vi "Analog Input Engine.vi"(5 "Main Engine Q":refnum<queue>, 7 "TCP Enigine Q":refnum<queue>, 8 "error in":errorcluster, 10 "Engine Name":string, 11 "Varient Data":variant) -> (0 "error out":errorcluster)   [LabVIEW 2024]
doc: "All Rights Reserved © 2023 SyncSols"
uses:
  Controls/Analog Input SM Data Cluster.ctl
  Analog Output/Controls/AIO Command Q Cluster.ctl
  Analog Output/Controls/AO Interface Data Cluster.ctl
  Analog Output/Controls/AO Channel Configuration Cluster.ctl
  Analog Output/Controls/AO Timing Cluster.ctl
  Main Engine/Controls/Main Engine JSON Command State.ctl
  TCP Engine/Controls/TCP Engine I&O  Interupt Cluster.ctl
  Host-DQMH/Configuration/Analog Input Single Channel Data--Cluster.ctl
  Host-DQMH/Configuration/Config-Channel Type.ctl
  Host-DQMH/Configuration/Channel Sub-Type.ctl
  Controls/Analog Input SM Cases.ctl
  Main Engine/Controls/Main Engine Engine No.Options.ctl
  Host-DQMH/Configuration/All Interface Data.ctl
  Host-DQMH/Configuration/DO Channel's.ctl
  Analog Output/Controls/AO JSON Data Cluster.ctl
  Main Engine/Controls/Main Engine Config Confirmation Cluster.ctl
  TCP Engine/TCP Engine.lvlib
  Host-DQMH/Configuration/Configuration.lvlib
panel:
  out "error out 4":errorcluster
  out "error out 3":errorcluster
  out "error out 2":errorcluster
  out "Configuration Data":T1[](array[typedef])
  in  "Data Cluster":T2={"TCP Engine Response Q"=refnum, "Main Engine Response Q"=refnum, "Command Q"=refnum, "Interupt Q"=refnum, "Stop Notifier"=refnum, "Start Notifier"=refnum, "Varient Data"=variant(string ""), "Engine Name"="", "Configuration Data"=[], "AI Task"="", "Single Sample?"=FALSE, "AI Config Data"={"Module Name"="", "AI Channel's Data"=[], "Analog Input Timing"={"samples per channel"=0, "sample mode"=0, "Sampling Rate"=0.0}}, "Configured Data's"={"Channel Names"=[], "Identification Names"=[]}, "AI Log File Path"=path ""} {"AI Config Data"."Analog Input Timing"."sample mode" items=["Finite Samples"=10178, "Continuous Samples"=10123, "Hardware Timed Single Point"=12522]}
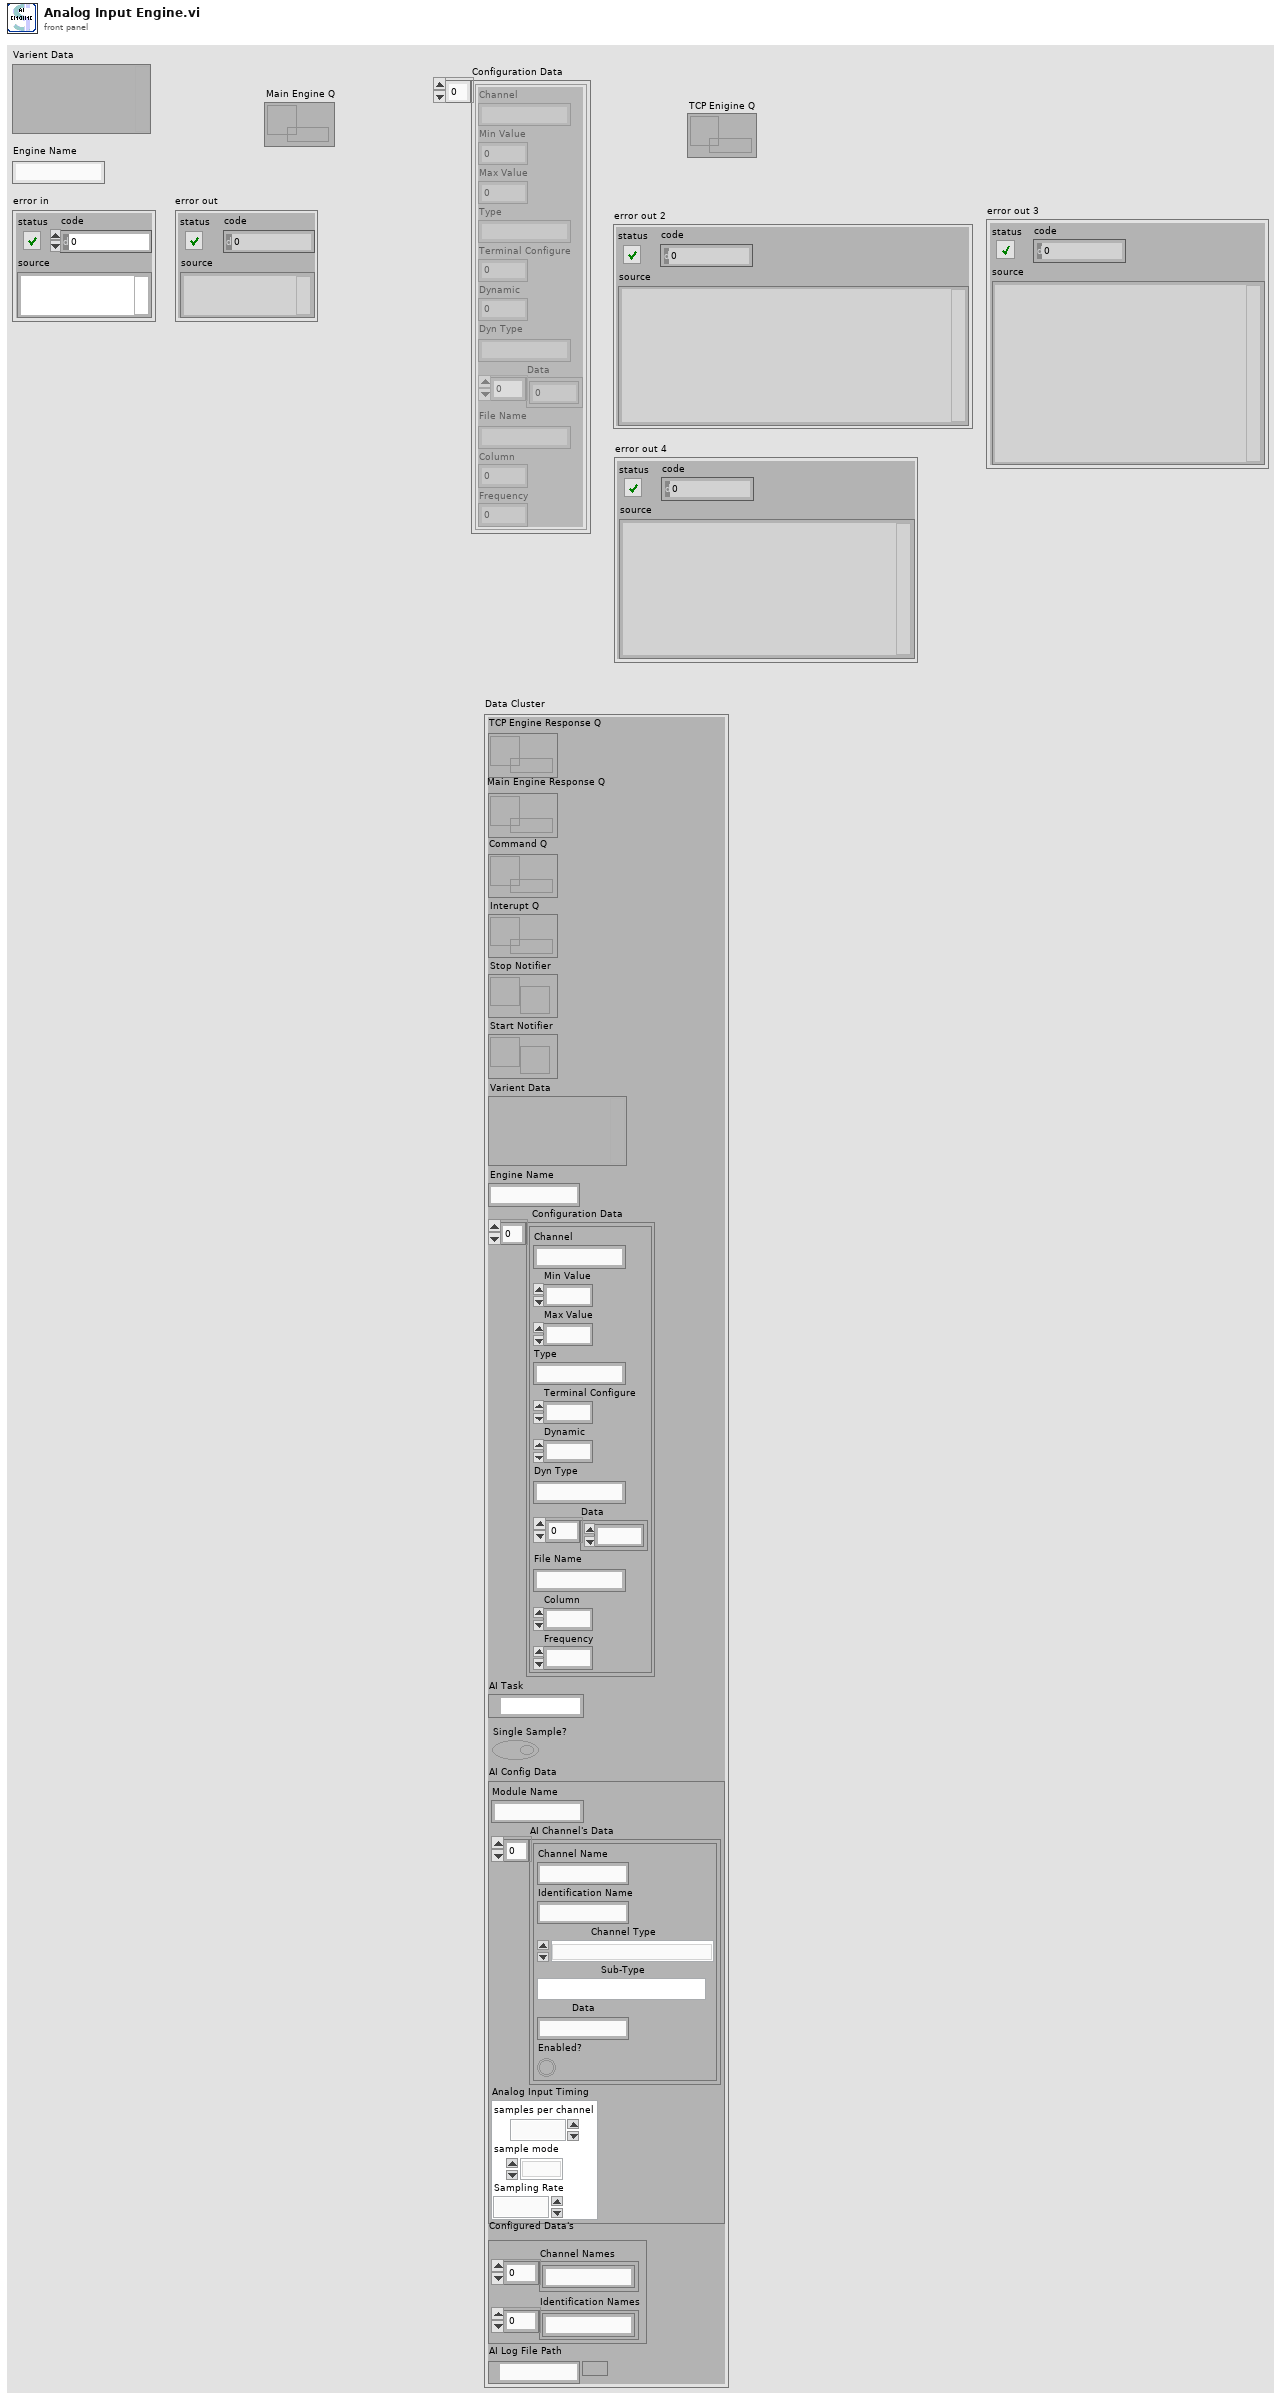
[diagram p1: front panel]
types:
  T1 = typedef "AO Channel Configuration Cluster.ctl" = cluster{"Channel":string, "Min Value":dbl, "Max Value":dbl, "Type":string, "Terminal Configure":u16, "Dynamic":u8, "Dyn Type":string, "Data":dbl[], "File Name":string, "Column":i32, "Frequency":dbl}
  T2 = typedef "Analog Input SM Data Cluster.ctl" = cluster{"TCP Engine Response Q":refnum<queue>, "Main Engine Response Q":refnum<queue>, "Command Q":refnum<queue>, "Interupt Q":refnum<queue>, "Stop Notifier":refnum<notifier>, "Start Notifier":refnum<notifier>, "Varient Data":variant, "Engine Name":string, "Configuration Data":T1[], "AI Task":refnum<k21>, "Single Sample?":bool, "AI Config Data":cluster{"Module Name":string, "AI Channel's Data":T3[], "Analog Input Timing":T6}, "Configured Data's":cluster{"Channel Names":string[], "Identification Names":string[]}, "AI Log File Path":path}
  T3 = typedef "Configuration.lvlib/Analog Input Single Channel Data--Cluster.ctl" = cluster{"Channel Name":string, "Identification Name":string, "Channel Type":T4, "Sub-Type":T5, "Data":string, "Enabled?":bool}
  T4 = typedef "Configuration.lvlib/Config-Channel Type.ctl" = enum16{"Voltage", "Current", "Thermocouple", "Acclerometer"}
  T5 = typedef "Configuration.lvlib/Channel Sub-Type.ctl" = enum16{"None", "Pressure", "Force"}
  T6 = typedef "AO Timing Cluster.ctl" = cluster{"samples per channel":i32, "sample mode":i32, "Sampling Rate":dbl}
  T7 = typedef "Analog Input SM Cases.ctl" = enum16{">Poll", ".........State Machine.........", ">Init", ">Error", ">Exit", "..........Analog Input..........", ">JSON to LV Data", ">Get Command", ">Configure", ">Start", ">Acquire", ">Stop"}
  T8 = typedef "TCP Engine.lvlib/TCP Engine I&O  Interupt Cluster.ctl" = cluster{" Stop":bool, "JSON Variant":variant}
  T9 = typedef "AIO Command Q Cluster.ctl" = cluster{"Interface":string, "Interface Data":T10, "Command State":T11}
  T10 = typedef "AO Interface Data Cluster.ctl" = cluster{"Command":string, "SubCmd":string, "Data":T1[], "Timing":T6}
  T11 = typedef "Main Engine JSON Command State.ctl" = enum16{"Configure", "Start", "Exit"}
  T12 = typedef "Main Engine Engine No.Options.ctl" = enum16{"Init", "Update", "Response", "Get"}
  T13 = typedef "Configuration.lvlib/All Interface Data.ctl" = cluster{"DI Config Data":T14, "DO Config Data":T14, "AI Config Data's":cluster{"Module Name":string, "AI Channel's Data":T3[], "Analog Input Timing":T6}[]}
  T14 = typedef "Configuration.lvlib/DO Channel's.ctl" = cluster{"Channel Name":string, "Identification Name":string, "Data":u8[], "Enabled?":bool}[]
  T15 = typedef "AO JSON Data Cluster.ctl" = cluster{"Interface":string, "Interface Data":T10}
  T16 = typedef "Main Engine Config Confirmation Cluster.ctl" = cluster{"Command":string, "Interface":string, "Status":string, "Board":string}
  T17 = cluster{"Module Name":string, "AI Channel's Data":T3[], "Analog Input Timing":T6}[]
  T18 = cluster{"Module Name":string, "AI Channel's Data":T3[], "Analog Input Timing":T6}
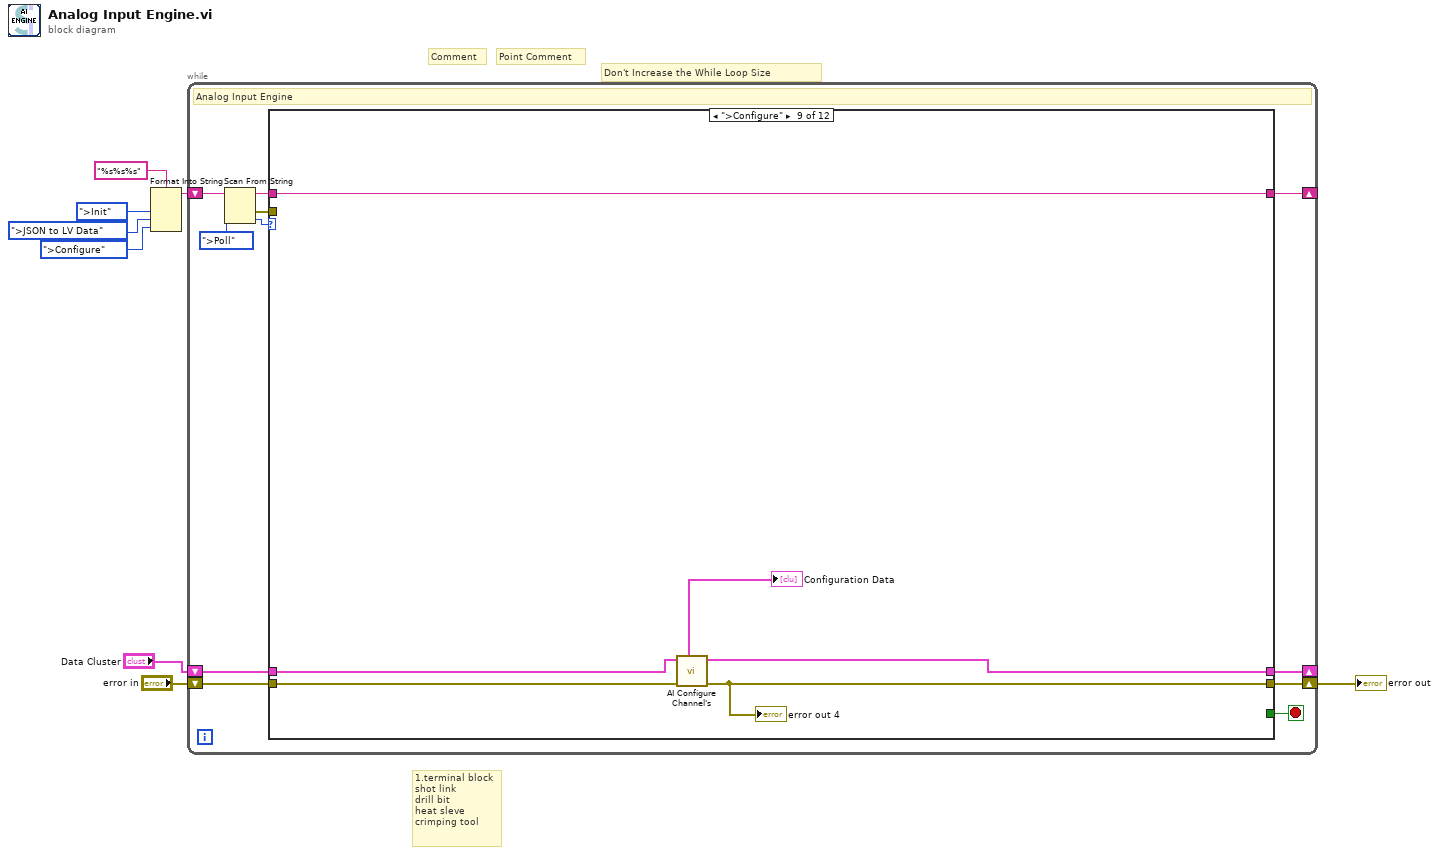
[diagram p0: block diagram]
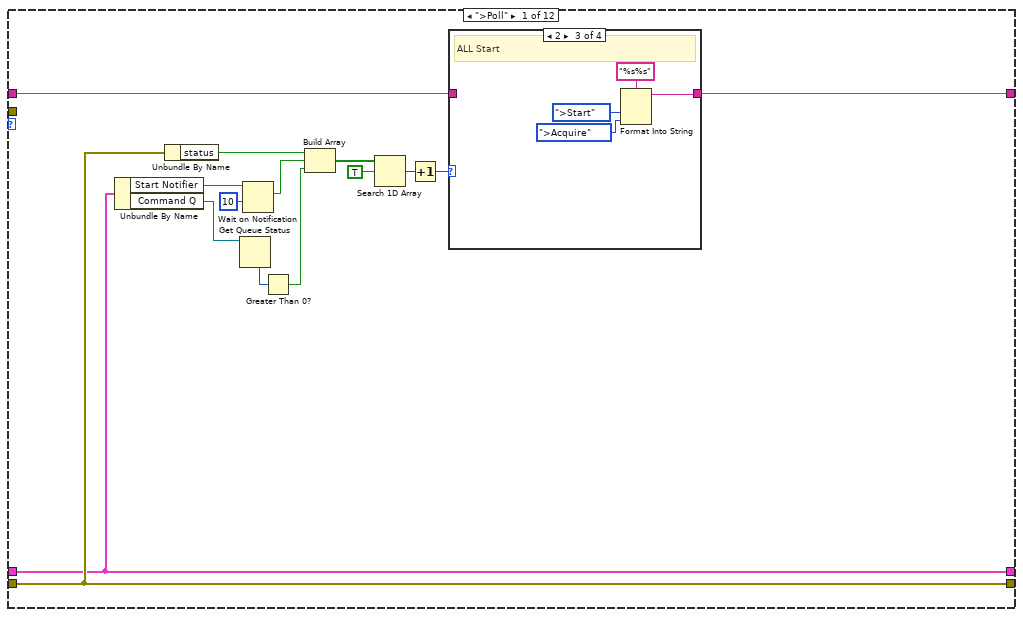
[diagram p2: hidden frame]
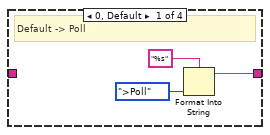
[diagram p3: hidden frame]
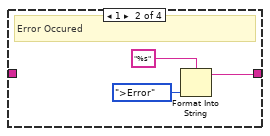
[diagram p4: hidden frame]
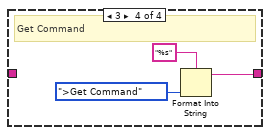
[diagram p5: hidden frame]
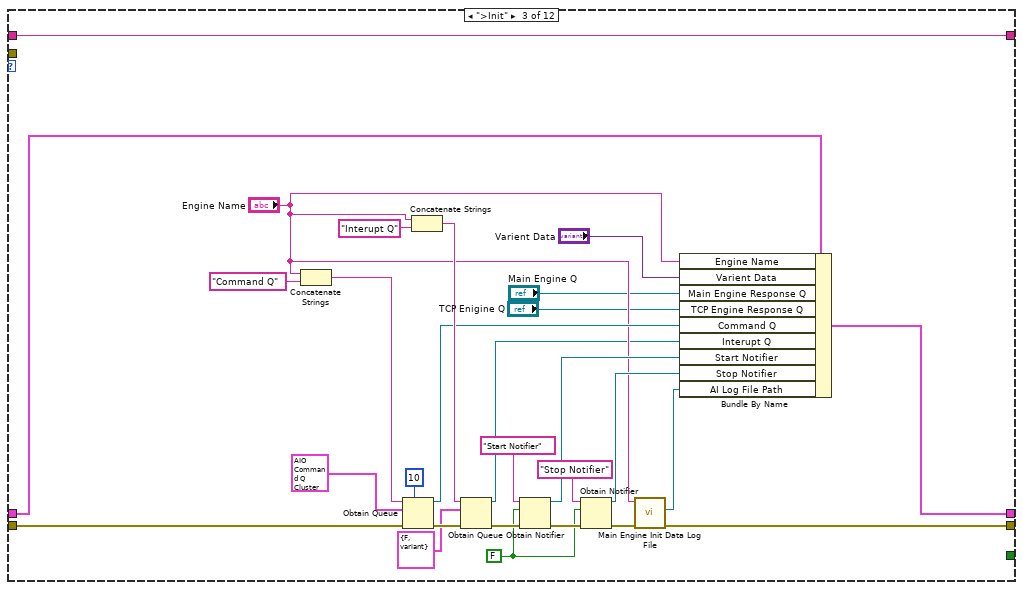
[diagram p7: hidden frame]
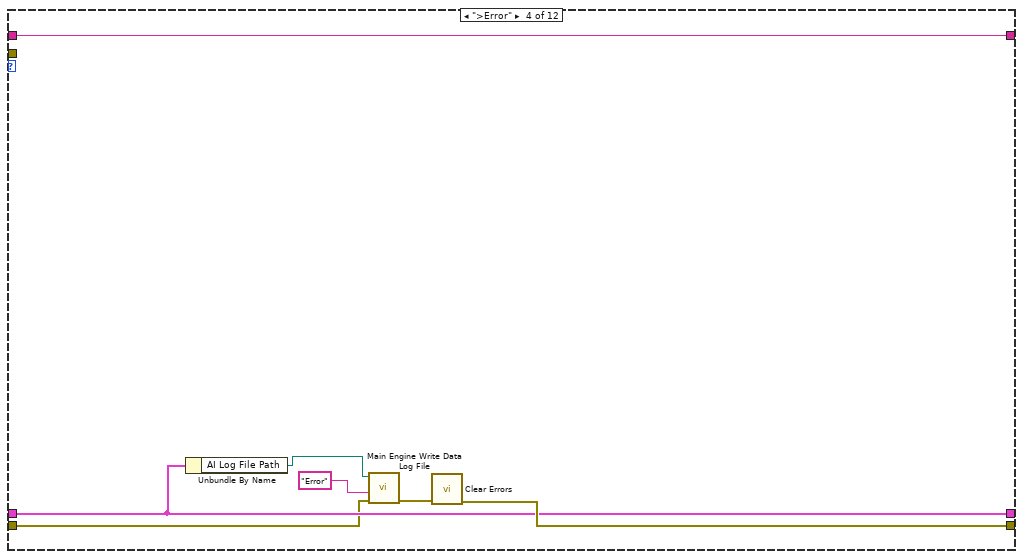
[diagram p8: hidden frame]
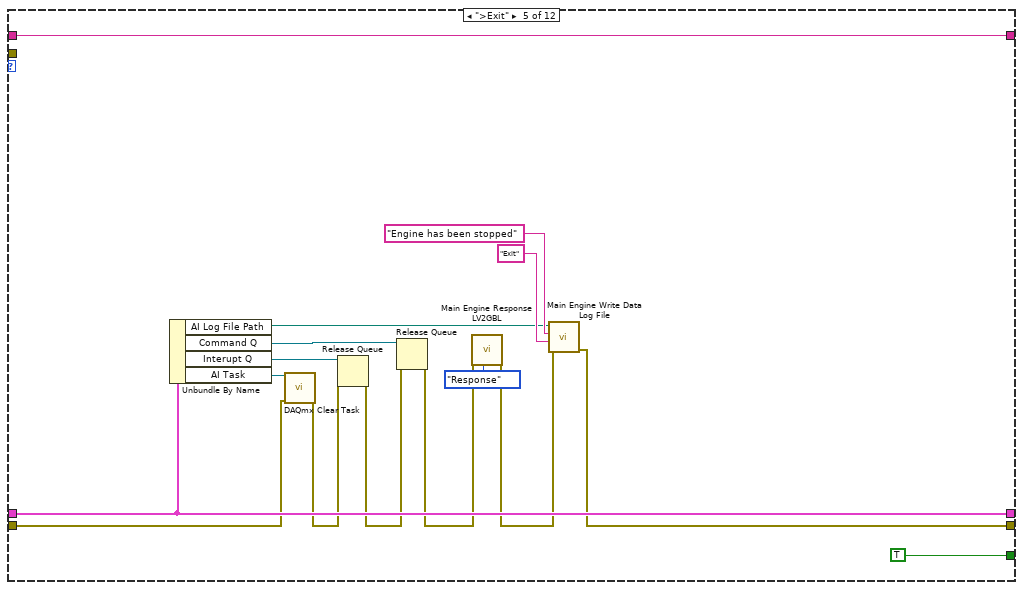
[diagram p9: hidden frame]
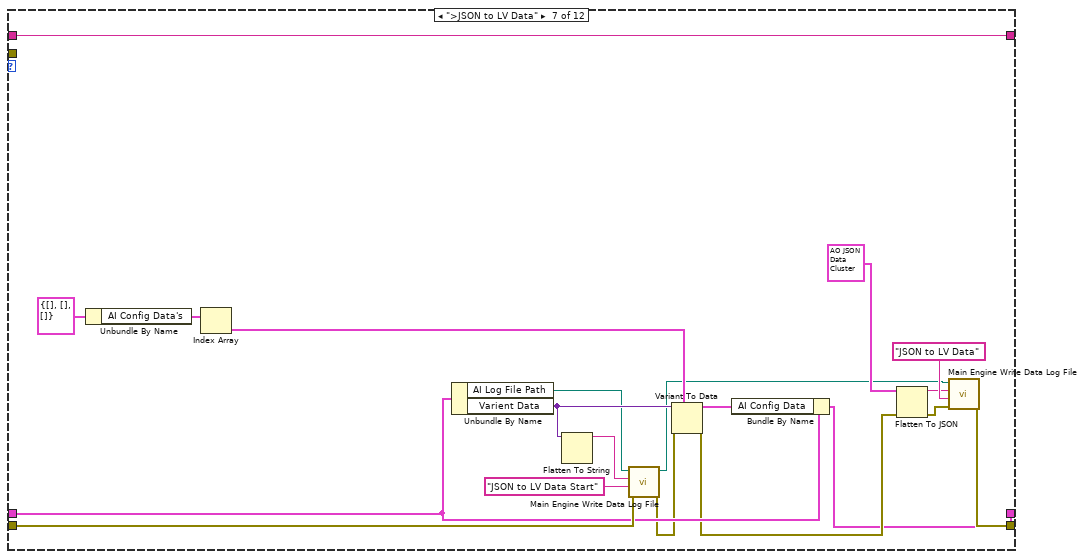
[diagram p11: hidden frame]
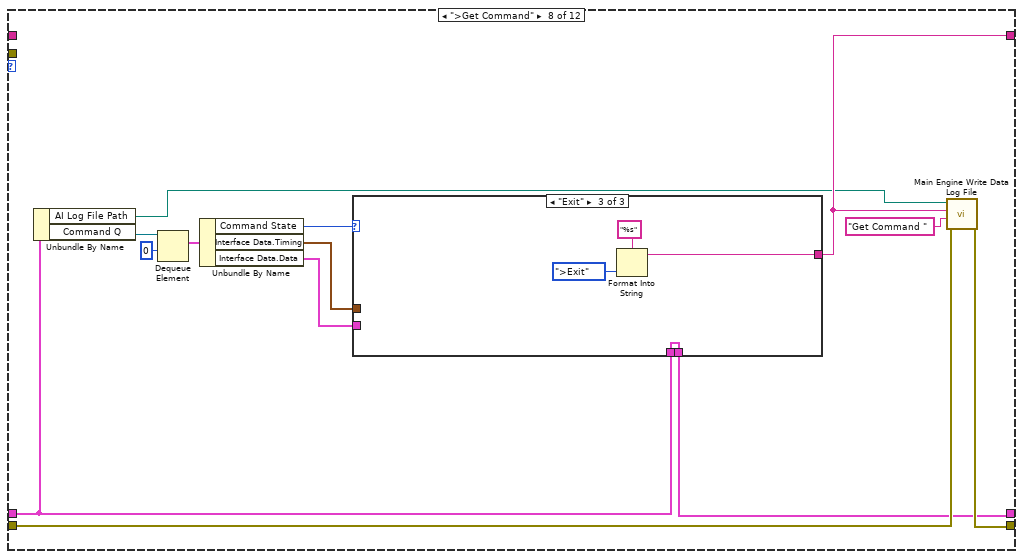
[diagram p12: hidden frame]
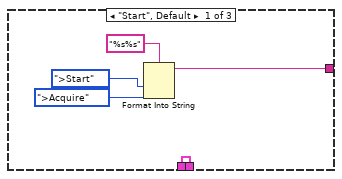
[diagram p13: hidden frame]
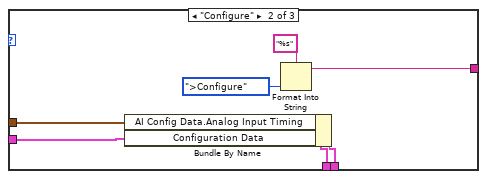
[diagram p14: hidden frame]
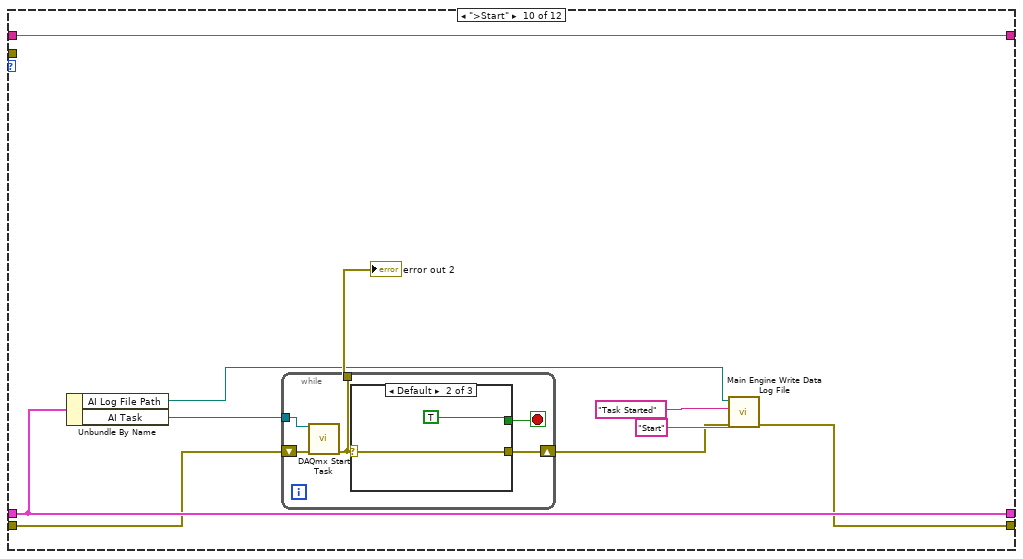
[diagram p15: hidden frame]
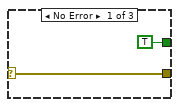
[diagram p16: hidden frame]
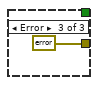
[diagram p17: hidden frame]
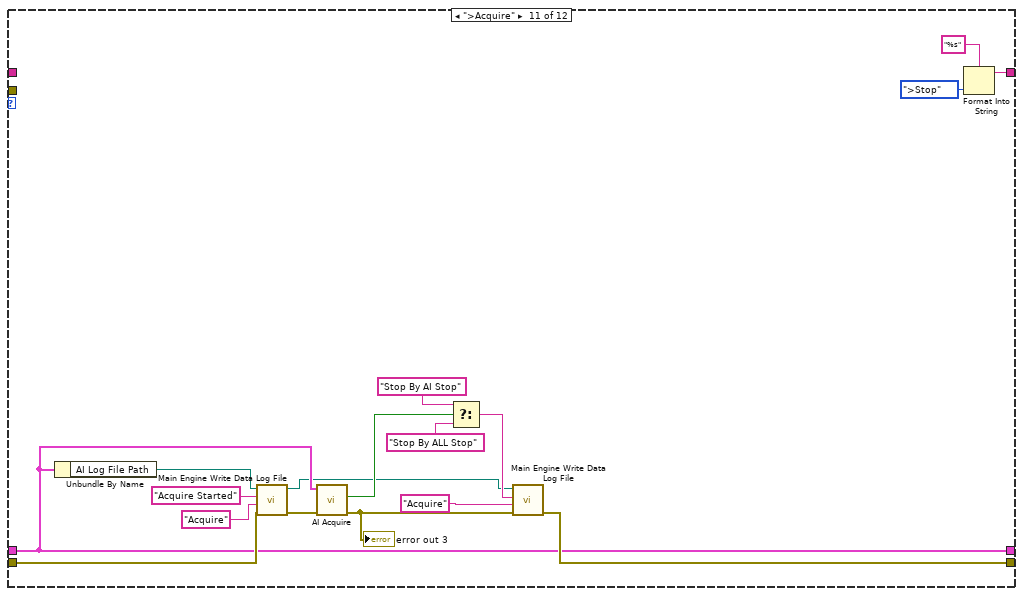
[diagram p18: hidden frame]
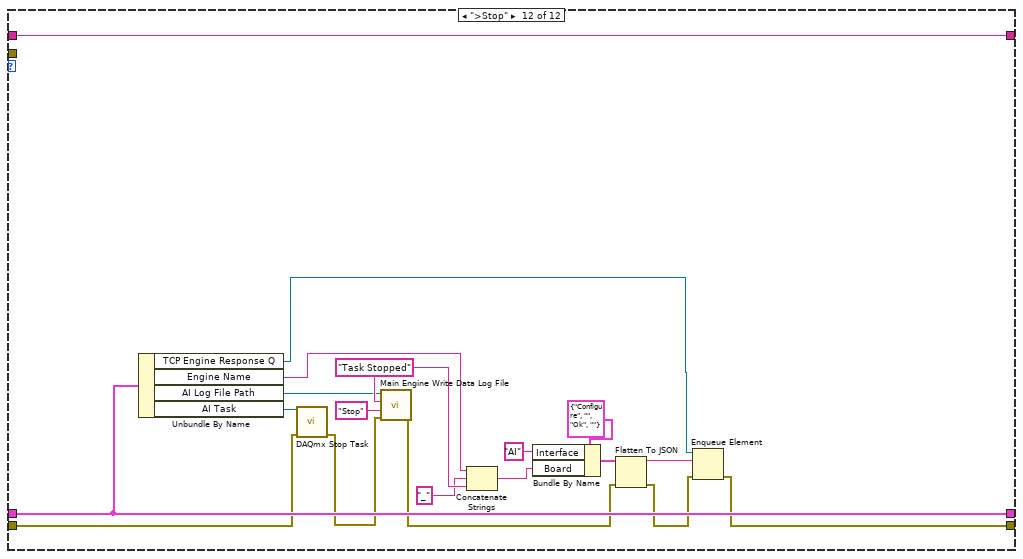
[diagram p19: hidden frame]
diagram:
  # "1.terminal block\nshot link\ndrill bit\nheat sleve\ncrimping tool"
  # "Don't Increase the While Loop Size"
  # "Point Comment"
  # "Comment"
  n1 = Format Into String(format string="%s%s%s", Analog_Input_SM_Cases.">Init" ("SM Cases Options"), Analog_Input_SM_Cases.">JSON to LV Data" ("input 2"), Analog_Input_SM_Cases.">Configure" ("input 3")) -> (resulting string=w7:string)  [unwired: 2 in, 1 out]
  n2 = while {
    shift-right: [w14] -> _
    shift-left: w7 -> [w19]
    shift-right: [w12] -> w4
    shift-left: "error in" -> [w13]
    shift-right: [w10] -> _
    shift-left: "Data Cluster" -> [w9]
    stop <- w11 stop-if-true
    # "Analog Input Engine"
    n3 = Scan From String(input string=w19, default 1=Analog_Input_SM_Cases.">Poll" ("SM Cases Options")) -> (remaining string=w15:string, error out=w17:errorcluster, output 1=w16:T7)  [unwired: 3 in, 1 out]
    n4 = case shown="\">Configure\"" w16 {
      tunnel: w17 -> [_ _ _ _ _ _ _ _ _ _ _ _]
      tunnel: w15 -> [w34 w50 w78 w85 w101 w104 w124 _ w159 w169 _ w215]
      tunnel: [w33 w50 w78 w85 w101 w104 w124 w130 w159 w169 w188 w215] -> w14
      tunnel: w13 -> [w32 w49 w56 w81 w91 w103 w121 w132 w157 w164 w196 w202]
      tunnel: [w32 w49 w61 w84 w95 w103 w120 w131 w154 w167 w192 w198] -> w12
      tunnel: [_ _ _ _ TRUE _ _ _ _ _ _ _] -> w11
      tunnel: [w26 w48 w66 w82 w99 w102 w113 w126 w156 w168 w185 w203] -> w10
      tunnel: w9 -> [w26 w48 w54 w82 w99 w102 w119 w127 w158 w168 w185 w203]
      frame ">Poll" {
        n5 = Unbundle By Name(w26) -> ("Start Notifier"=w25:refnum<notifier>, "Command Q"=w23:refnum<queue>)
        n6 = Unbundle By Name(w32) -> ("status"=w31:bool)
        n7 = Get Queue Status(queue=w23) -> (# elements in queue=w21:i32)  [unwired: 2 in, 7 out]
        n8 = Wait on Notification(notifier=w25, timeout in ms (-1)=10) -> (notification=w22:bool)  [unwired: 2 in, 3 out]
        n9 = Greater Than 0?(x=w21) -> (x > 0?=w20:bool)
        n10 = Build Array(w31, w22, w20) -> (w30:bool[])
        n11 = Search 1D Array(1D array=w30, element=TRUE) -> (index of element=w28:i32)  [unwired: 1 in]
        n12 = Increment(x=w28) -> (x+1=w27:i32)
        n13 = case shown="2" w27 {
          tunnel: w34 -> [_ _ _ _]
          tunnel: [w35 w38 w42 w45] -> w33
          frame 0, Default {
            # "Default -> Poll"
            n14 = Format Into String(format string="%s", Analog_Input_SM_Cases.">Poll" ("SM Cases Options")) -> (resulting string=w35:string)  [unwired: 2 in, 1 out]
          }
          frame 1 {
            # "Error Occured"
            n15 = Format Into String(format string="%s", Analog_Input_SM_Cases.">Error" ("SM Cases Options")) -> (resulting string=w38:string)  [unwired: 2 in, 1 out]
          }
          frame 2 {
            # "ALL Start"
            n16 = Format Into String(format string="%s%s", Analog_Input_SM_Cases.">Start" ("SM Cases Options"), Analog_Input_SM_Cases.">Acquire" ("input 2")) -> (resulting string=w42:string)  [unwired: 2 in, 1 out]
          }
          frame 3 {
            # "Get Command"
            n17 = Format Into String(format string="%s", Analog_Input_SM_Cases.">Get Command" ("SM Cases Options")) -> (resulting string=w45:string)  [unwired: 2 in, 1 out]
          }
        }
      }
      frame ".........State Machine........." {
      }
      frame ">Init" {
        w67 = FALSE
        n18 = Concatenate Strings("Engine Name", "Command Q" ("name (unnamed)")) -> (w75:string)
        n19 = Obtain Queue(max queue size (-1, unlimited)=10, name (unnamed)=w75, element data type=T9 {"Interface"="AIO", "Interface Data"={"Command"="Configure", "SubCmd"="AO", "Data"=[], "Timing"={"samples per channel"=1000, "sample mode"=10178, "Sampling Rate"=1000.0}}, "Command State"=enum."Configure"} ("AIO Config Cluster"), error in (no error)=w56) -> (queue out=w63:refnum<queue>, error out=w73:errorcluster)  [unwired: 1 in, 1 out]
        n20 = Concatenate Strings("Engine Name", "Interupt Q" ("name (unnamed)")) -> (w72:string)
        n21 = Obtain Queue(name (unnamed)=w72, element data type=T8 {" Stop"=FALSE, "JSON Variant"=variant(string "")} ("I/O  Interupt Cluster"), error in (no error)=w73) -> (queue out=w58:refnum<queue>, error out=w71:errorcluster)  [unwired: 2 in, 1 out]
        n22 = Obtain Notifier(name (unnamed)="Start Notifier", notification data type=w67, error in (no error)=w71) -> (notifier out=w64:refnum<notifier>, error out=w70:errorcluster)  [unwired: 1 in, 1 out]
        n23 = Obtain Notifier(name (unnamed)="Stop Notifier", notification data type=w67, error in (no error)=w70) -> (notifier out=w65:refnum<notifier>, error out=w62:errorcluster)  [unwired: 1 in, 1 out]
        n24 = call "Main Engine Init Data Log File.vi"("error in"=w62, "Engine Name"="Engine Name") -> ("error out"=w61:errorcluster, "Log File Path"=w51:path)  [unwired: 8 in]
        n25 = Bundle By Name(cluster=w54, "Engine Name"="Engine Name", "Varient Data"="Varient Data", "Main Engine Response Q"="Main Engine Q", "TCP Engine Response Q"="TCP Enigine Q", "Command Q"=w63, "Interupt Q"=w58, "Start Notifier"=w64, "Stop Notifier"=w65, "AI Log File Path"=w51) -> (w66:T2)
      }
      frame ">Error" {
        n26 = Unbundle By Name(w82) -> ("AI Log File Path"=w79:path)
        n27 = call "Main Engine Write Data Log File.vi"("error in"=w81, "State"="Error" ("Input Data"), "Log file path In"=w79) -> ("error out"=w80:errorcluster)  [unwired: 7 in, 1 out]
        n28 = call <vilib>:"Clear Errors.vi"("error in (no error)"=w80) -> ("error out"=w84:errorcluster)  [unwired: 5 in, 1 out]
      }
      frame ">Exit" {
        n29 = Unbundle By Name(w99) -> ("AI Log File Path"=w86:path, "Command Q"=w97:refnum<queue>, "Interupt Q"=w98:refnum<queue>, "AI Task"=w90:refnum<k21>)
        n30 = call <vilib>:"DAQmx Clear Task.vi"("task in"=w90, "error in"=w91) -> ("error out"=w92:errorcluster)  [unwired: 13 in]
        n31 = Release Queue(queue=w98, error in (no error)=w92) -> (error out=w96:errorcluster)  [unwired: 1 in, 2 out]
        n32 = Release Queue(queue=w97, error in (no error)=w96) -> (error out=w89:errorcluster)  [unwired: 1 in, 2 out]
        n33 = call "Main Engine Response LV2GBL.vi"("Options"=Main_Engine_Engine_No.Options."Response", "error in"=w89) -> ("error out"=w88:errorcluster)  [unwired: 7 in, 2 out]
        n34 = call "Main Engine Write Data Log File.vi"("error in"=w88, "State"="Exit", "Input Data"="Engine has been stopped", "Log file path In"=w86) -> ("error out"=w95:errorcluster)  [unwired: 6 in, 1 out]
      }
      frame "..........Analog Input.........." {
      }
      frame ">JSON to LV Data" {
        n35 = Unbundle By Name(T13 {"DI Config Data"=[], "DO Config Data"=[], "AI Config Data's"=[]} ("Interface Data")) -> ("AI Config Data's"=w109:T17)
        n36 = Index Array(array=w109) -> (element=w108:T18)  [unwired: 1 in]
        n37 = Unbundle By Name(w119) -> ("AI Log File Path"=w106:path, "Varient Data"=w112:variant)
        n38 = Flatten To String(anything=w112) -> (data string=w114:string)  [unwired: 3 in, 2 out]
        n39 = call "Main Engine Write Data Log File.vi"("error in"=w121, "State"="JSON to LV Data Start", "Input Data"=w114, "Log file path In"=w106) -> ("error out"=w115:errorcluster, "Log File Path Out"=w105:path)  [unwired: 6 in]
        n40 = Variant To Data(error in=w115, type=w108, Variant=w112) -> (data=w107:T18, error out=w117:errorcluster)
        n41 = Bundle By Name(cluster=w119, "AI Config Data"=w107) -> (w113:T2)
        n42 = Flatten To JSON(anything=T15 {"Interface"="AIO", "Interface Data"={"Command"="Configure", "SubCmd"="AO", "Data"=[], "Timing"={"samples per channel"=0, "sample mode"=10178, "Sampling Rate"=0.0}}} ("AO JSON Data Cluster"), error in (no error)=w117) -> (JSON string=w118:string, 11:w116:errorcluster)  [unwired: 1 in]
        n43 = call "Main Engine Write Data Log File.vi"("error in"=w116, "State"="JSON to LV Data", "Input Data"=w118, "Log file path In"=w105) -> ("error out"=w120:errorcluster)  [unwired: 6 in, 1 out]
      }
      frame ">Get Command" {
        n44 = Unbundle By Name(w127) -> ("AI Log File Path"=w125:path, "Command Q"=w137:refnum<queue>)
        n45 = Dequeue Element(queue=w137, timeout in ms (-1)=0) -> (element=w135:T9)  [unwired: 1 in, 3 out]
        n46 = Unbundle By Name(w135) -> ("Command State"=w134:T11, "Interface Data.Timing"=w129:T6, "Interface Data.Data"=w128:T1[])
        n47 = case shown="\"Exit\"" w134 {
          tunnel: [w141 w148 w152] -> w130
          tunnel: w129 -> [_ w146 _]
          tunnel: w128 -> [_ w145 _]
          tunnel: w127 -> [w138 w144 w150]
          tunnel: [w138 w143 w150] -> w126
          frame "Start", Default {
            n48 = Format Into String(format string="%s%s", Analog_Input_SM_Cases.">Start" ("SM Cases Options"), Analog_Input_SM_Cases.">Acquire" ("SM Cases Options")) -> (resulting string=w141:string)  [unwired: 2 in, 1 out]
          }
          frame "Configure" {
            n49 = Bundle By Name(cluster=w144, "AI Config Data.Analog Input Timing"=w146, "Configuration Data"=w145) -> (w143:T2)
            n50 = Format Into String(format string="%s", Analog_Input_SM_Cases.">Configure" ("SM Cases Options")) -> (resulting string=w148:string)  [unwired: 2 in, 1 out]
          }
          frame "Exit" {
            n51 = Format Into String(format string="%s", Analog_Input_SM_Cases.">Exit" ("SM Cases Options")) -> (resulting string=w152:string)  [unwired: 2 in, 1 out]
          }
        }
        n52 = call "Main Engine Write Data Log File.vi"("error in"=w132, "State"="Get Command ", "Input Data"=w130, "Log file path In"=w125) -> ("error out"=w131:errorcluster)  [unwired: 6 in, 1 out]
      }
      frame ">Configure" {
        n53 = call "AI Configure Channel's.vi"("error in (no error)"=w157, "Data Cluster in"=w158) -> ("error out"=w154:errorcluster, "Data Cluster out"=w156:T2, "Configuration Data"=→"Configuration Data":T1[])  [unwired: 7 in]
        "error out 4" <- w154
      }
      frame ">Start" {
        n54 = Unbundle By Name(w168) -> ("AI Log File Path"=w160:path, "AI Task"=w163:refnum<k21>)
        n55 = while {
          tunnel: w163 -> [w173]
          shift-right: [w172] -> w162
          shift-left: w164 -> [w174]
          tunnel: [w170] -> w161
          stop <- w171 stop-if-true
          n56 = call <vilib>:"DAQmx Start Task.vi"("task/channels in"=w173, "error in"=w174) -> ("error out"=w170:errorcluster)  [unwired: 12 in, 1 out]
          n57 = case shown="Default" w170 {
            selector: w170 -> [w176 w178 _]
            tunnel: [w176 w178 errorcluster {"status"=FALSE, "code"=0, "source"=""} ("error IO")] -> w172
            tunnel: [TRUE TRUE _] -> w171
            frame No Error {
            }
            frame Default {
            }
            frame Error {
            }
          }
        }
        "error out 2" <- w161
        n58 = call "Main Engine Write Data Log File.vi"("error in"=w162, "State"="Start", "Input Data"="Task Started", "Log file path In"=w160) -> ("error out"=w167:errorcluster)  [unwired: 6 in, 1 out]
      }
      frame ">Acquire" {
        n59 = Unbundle By Name(w185) -> ("AI Log File Path"=w181:path)
        n60 = call "Main Engine Write Data Log File.vi"("error in"=w196, "State"="Acquire", "Input Data"="Acquire Started", "Log file path In"=w181) -> ("error out"=w184:errorcluster, "Log File Path Out"=w180:path)  [unwired: 6 in]
        n61 = call "AI Acquire.vi"("error in (no error)"=w184, "Data Cluster in"=w185) -> ("error out"=w182:errorcluster, "Stop"=w183:bool)  [unwired: 8 in]
        "error out 3" <- w182
        n62 = Select(t="Stop By AI Stop" ("State"), s=w183, f="Stop By ALL Stop" ("State")) -> (s? t:f=w189:string)
        n63 = call "Main Engine Write Data Log File.vi"("error in"=w182, "State"="Acquire", "Input Data"=w189, "Log file path In"=w180) -> ("error out"=w192:errorcluster)  [unwired: 6 in, 1 out]
        n64 = Format Into String(format string="%s", Analog_Input_SM_Cases.">Stop" ("input 1")) -> (resulting string=w188:string)  [unwired: 2 in, 1 out]
      }
      frame ">Stop" {
        w207 = "Task Stopped" ("Input Data")
        n65 = Unbundle By Name(w203) -> ("TCP Engine Response Q"=w210:refnum<queue>, "Engine Name"=w209:string, "AI Log File Path"=w197:path, "AI Task"=w214:refnum<k21>)
        n66 = call <vilib>:"DAQmx Stop Task.vi"("task/channels in"=w214, "error in"=w202) -> ("error out"=w201:errorcluster)  [unwired: 12 in, 1 out]
        n67 = call "Main Engine Write Data Log File.vi"("error in"=w201, "State"="Stop", "Input Data"=w207, "Log file path In"=w197) -> ("error out"=w200:errorcluster)  [unwired: 6 in, 1 out]
        n68 = Concatenate Strings(w209, "_", w207) -> (w212:string)
        n69 = Bundle By Name(cluster=T16 {"Command"="Configure", "Interface"="", "Status"="Ok", "Board"=""}, "Interface"="AI" ("SubCmd"), "Board"=w212) -> (w211:T16)
        n70 = Flatten To JSON(anything=w211, error in (no error)=w200) -> (JSON string=w213:string, 11:w199:errorcluster)  [unwired: 1 in]
        n71 = Enqueue Element(queue=w210, element=w213, error in (no error)=w199) -> (error out=w198:errorcluster)  [unwired: 1 in, 2 out]
      }
    }
  }
  "error out" <- w4
